vi "Device_Calibration.vi"(10 "PEU":refnum<class "PEU.lvclass">, 11 "E5071C":refnum<class "E5071C.lvclass">) -> ()   [LabVIEW 2020]
uses:
  Driver/E5071C/E5071C/E5071C.lvclass
  Driver/PEU/PEU/PEU.lvclass
panel:
  in  "TP1 - TP4":bool
  out ":SENS":i32
  in  "TP1 - TP3":bool
  in  "Next Button":bool
  in  "设置":bool
  in  "扫描点数":dbl=1001.0 caption="扫描点数\nSweep Points" min=2.0 max=1601.0 format="%#_6f"
  in  "中频带宽":dbl=70.0 caption="中频带宽\nIFBW" min=0.01 max=700.0 format="%#_6f kHz"
  in  "终止频率":dbl=20.0 caption="终止频率\nStop Frequency" min=0.0003 max=20.0 format="%#_6f GHz"
  in  "开始频率":dbl=300.0 caption="开始频率\nStart Frequency" min=300.0 max=20000000.0 format="%#_6f kHz"
  # "E5071C设置/校准"
  # "校准"
  # "参数设置"
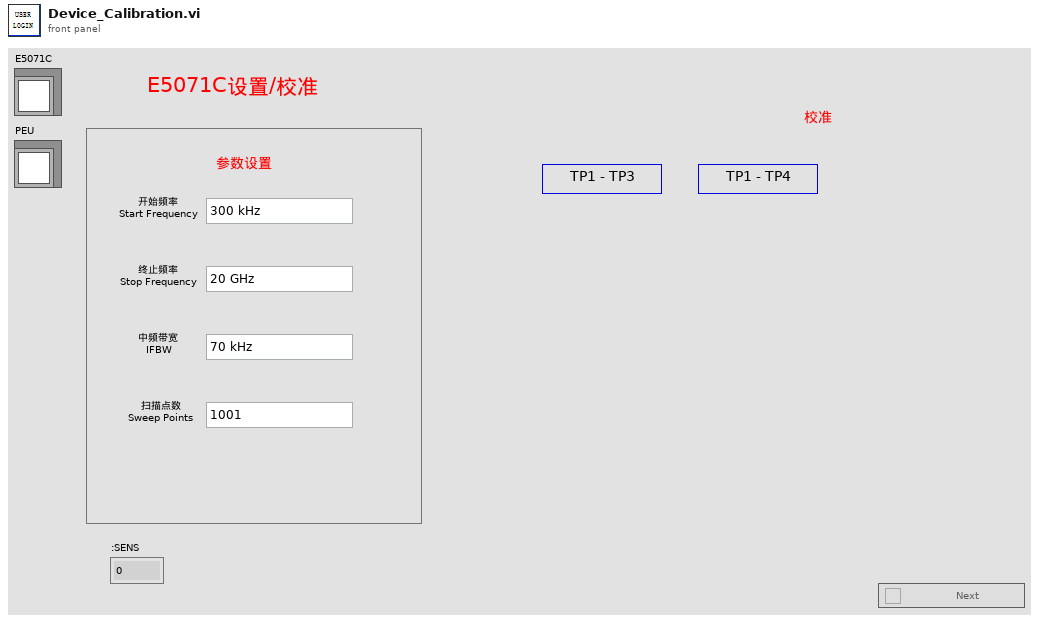
[diagram p1: front panel]
types:
  T1 = enum8{"Enabled", "Disabled", "Disabled and Grayed Out"}
  T2 = cluster{"E5071C":refnum<class "E5071C.lvclass">, "TP":string, "TPs":string[], "PEU":refnum<class "PEU.lvclass">}
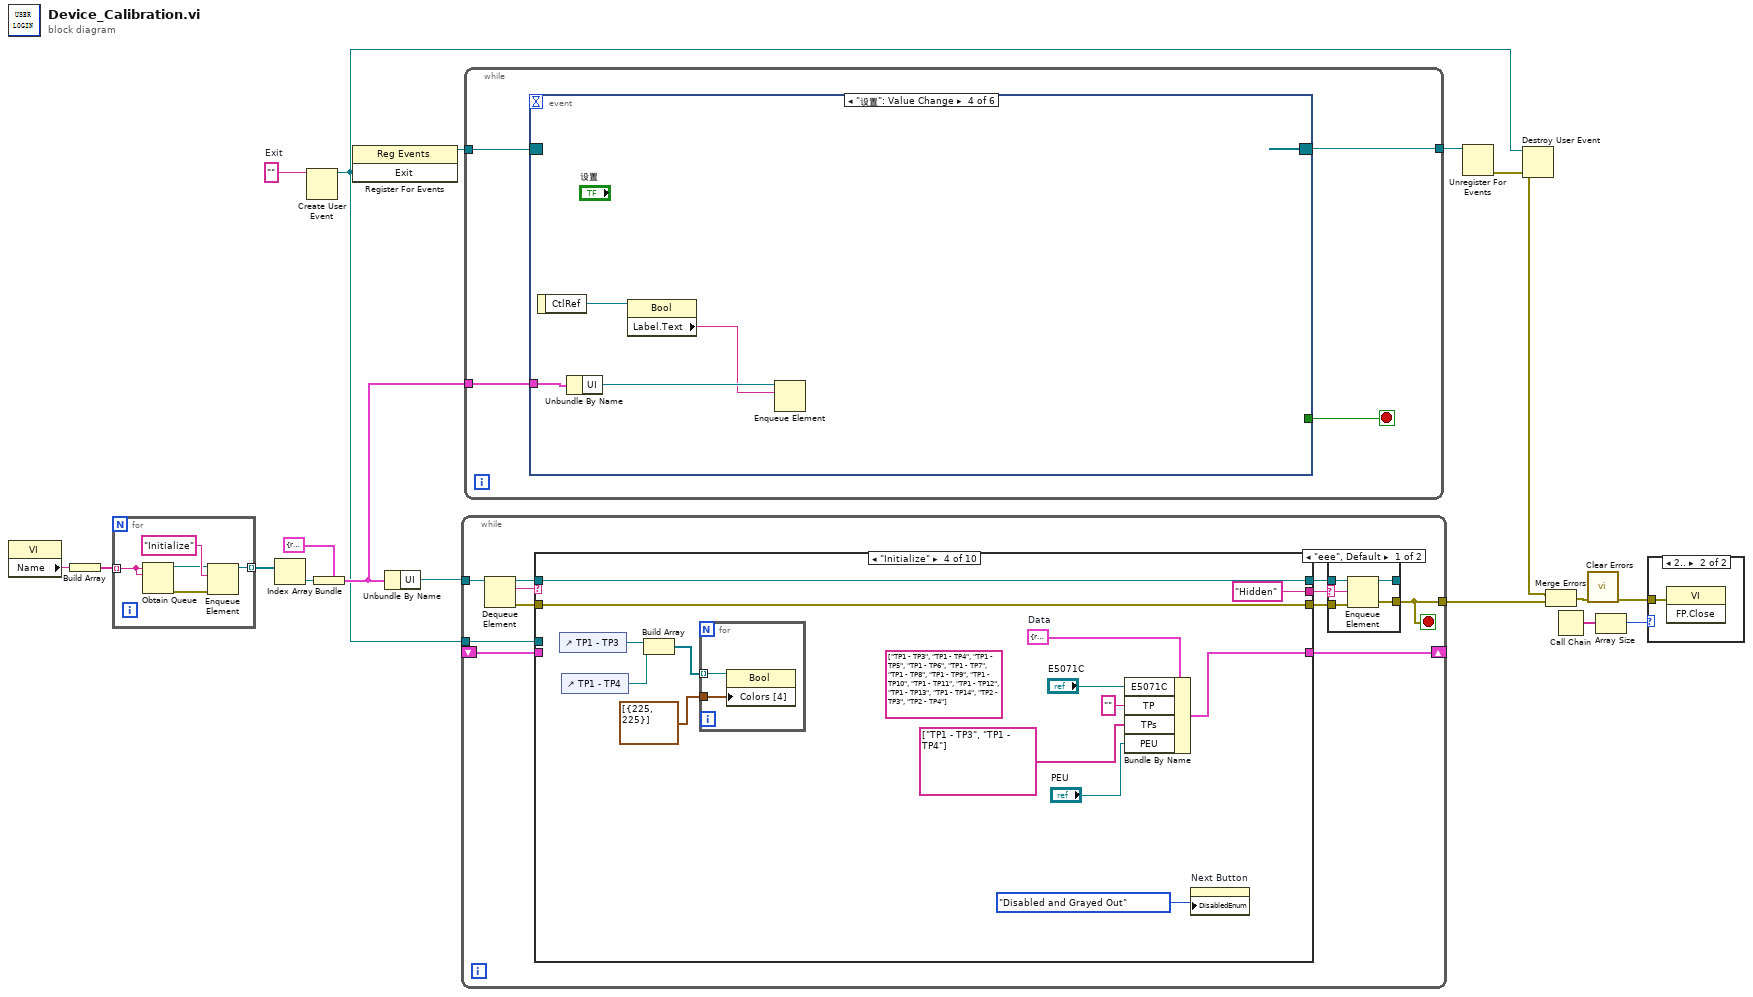
[diagram p0: block diagram]
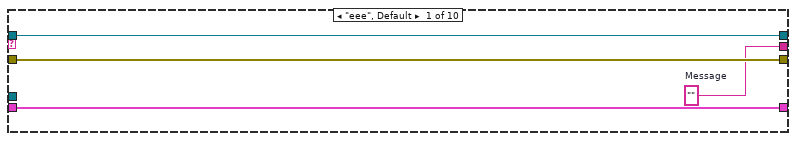
[diagram p4: hidden frame]
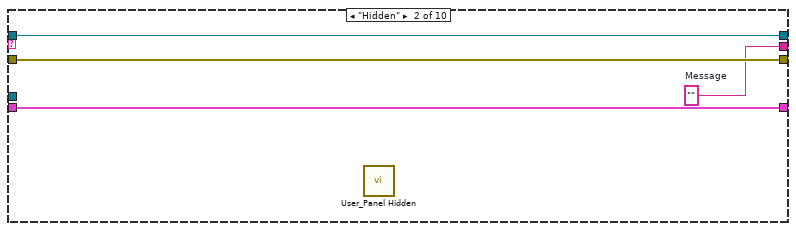
[diagram p5: hidden frame]
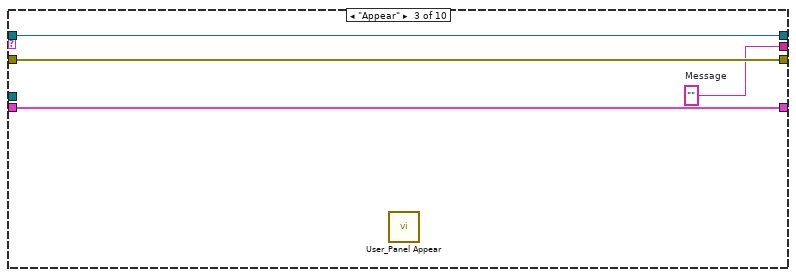
[diagram p6: hidden frame]
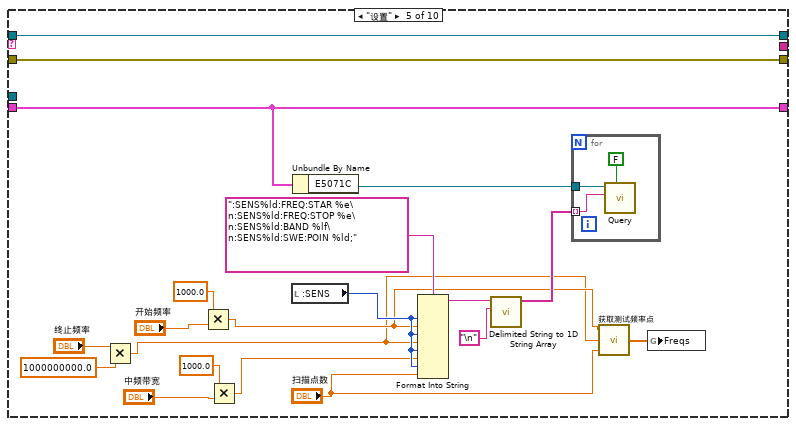
[diagram p7: hidden frame]
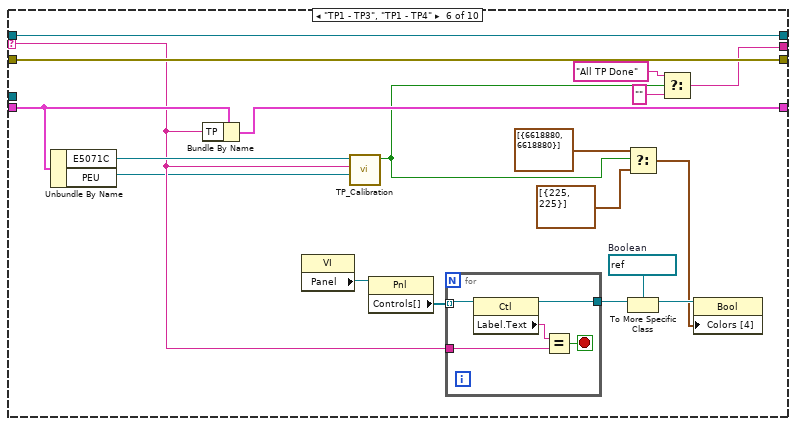
[diagram p8: hidden frame]
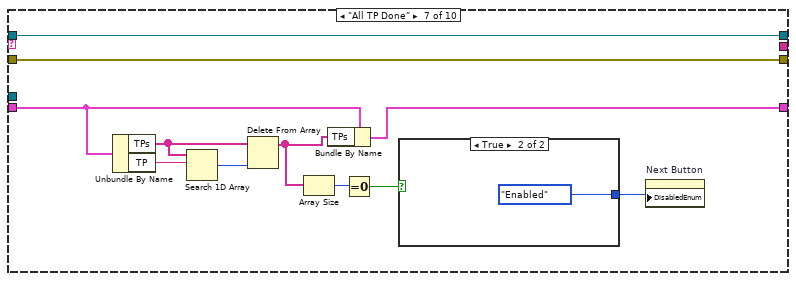
[diagram p9: hidden frame]
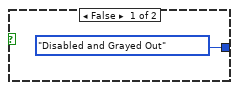
[diagram p10: hidden frame]
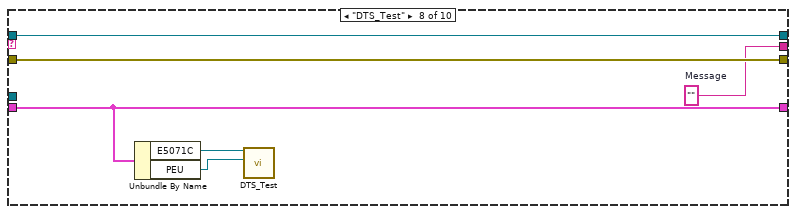
[diagram p11: hidden frame]
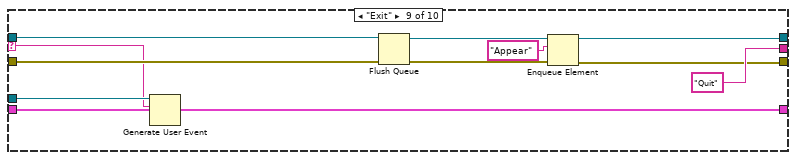
[diagram p12: hidden frame]
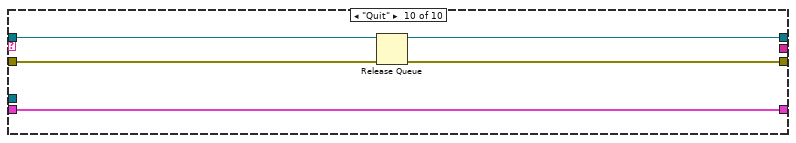
[diagram p13: hidden frame]
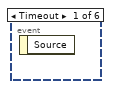
[diagram p14: hidden frame]
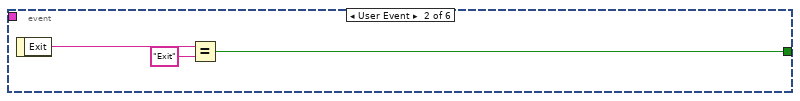
[diagram p15: hidden frame]
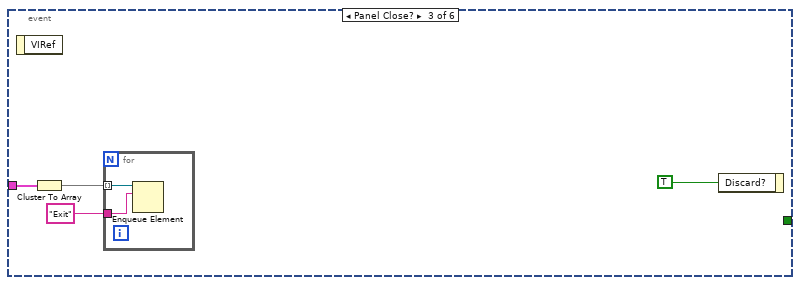
[diagram p16: hidden frame]
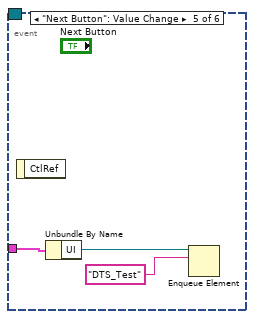
[diagram p17: hidden frame]
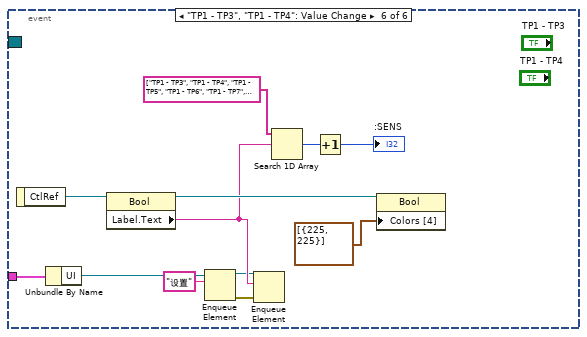
[diagram p18: hidden frame]
diagram:
  w7 = ""  # Exit
  n1 = property class="VI"() -> ("Name"=w17:string)  [unwired: 2 in, 2 out]
  n2 = Build Array(w17) -> (w18:string[])
  n3 = for {
    tunnel: w18 -> [w19] mode=indexing
    tunnel: [w20] -> w12 mode=indexing
    n4 = Obtain Queue(name (unnamed)=w19, element data type=w19) -> (queue out=w22:refnum<queue>, error out=w21:errorcluster)  [unwired: 3 in, 1 out]
    n5 = Enqueue Element(queue=w22, element="Initialize" ("元素"), error in (no error)=w21) -> (queue out=w20:refnum<queue>)  [unwired: 1 in, 2 out]
  }
  n6 = Index Array(array=w12) -> (element=w15:refnum<queue>)  [unwired: 1 in]
  n7 = Create User Event(user event datatype=w7) -> (user event=w11:refnum<user-event>)  [unwired: 1 in, 1 out]
  n8 = Bundle(cluster=cluster{"UI":refnum<queue>} {"UI"=refnum}, "UI"=w15) -> (w16:cluster{"UI":refnum<queue>})
  n9 = register-events(w11) -> (reference out=w8:refnum<event-registration>)  [unwired: 2 in, 1 out]
  n10 = Unbundle By Name(w16) -> ("UI"=w13:refnum<queue>)
  n11 = while {
    tunnel: w13 -> [w34]
    tunnel: [w24] -> w1
    shift-right: [w28] -> _
    shift-left: _ -> [w27]
    tunnel: w11 -> [w26]
    stop <- w24 stop-if-true
    n12 = Dequeue Element(queue=w34) -> (queue out=w33:refnum<queue>, element=w25:string, error out=w30:errorcluster)  [unwired: 2 in, 1 out]
    n13 = case shown="\"Initialize\"" w25 {
      selector: w25 -> [_ _ _ _ _ w99 _ _ w141 _]
      tunnel: w33 -> [w45 w49 w53 w67 w89 w111 w127 w135 w144 w150]
      tunnel: [w45 w49 w53 w67 w89 w111 w127 w135 w136 w150] -> w32
      tunnel: [w44 w48 w52 w66 w88 w110 w126 w134 w137 w147] -> w31
      tunnel: w30 -> [w44 w48 w52 w66 w88 w110 w126 w134 w143 w149]
      tunnel: [w43 w47 w51 "Hidden" ("Message") _ w95 _ w133 "Quit" ("Message") _] -> w29
      tunnel: [w42 w46 w50 w63 w87 w98 w119 w132 w146 w148] -> w28
      tunnel: w27 -> [w42 w46 w50 _ w87 w100 w121 w132 w146 w148]
      tunnel: w26 -> [_ _ _ _ _ _ _ _ w142 _]
      frame "eee", Default {
        w43 = ""  # Message
      }
      frame "Hidden" {
        w47 = ""  # Message
        n14 = call "User_Panel Hidden.vi"() -> ()  [unwired: 11 in, 1 out]
      }
      frame "Appear" {
        w51 = ""  # Message
        n15 = call "User_Panel Appear.vi"() -> ()  [unwired: 11 in, 1 out]
      }
      frame "Initialize" {
        (unwired) string[] ["TP1 - TP3", "TP1 - TP4", "TP1 - TP5", "TP1 - TP6", "TP1 - TP7", "TP1 - TP8", "TP1 - TP9", "TP1 - TP10", "TP1 - TP11", "TP1 - TP12", "TP1 - TP13", "TP1 - TP14", "TP2 - TP3", "TP2 - TP4"]
        w65 = T2 {"E5071C"=refnum, "TP"="", "TPs"=["TP1 - TP3", "TP1 - TP4", "TP1 - TP5", "TP1 - TP6", "TP1 - TP7", "TP1 - TP8", "TP1 - TP9", "TP1 - TP10", "TP1 - TP11", "TP1 - TP12", "TP1 - TP13", "TP1 - TP14", "TP2 - TP3", "TP2 - TP4"], "PEU"=refnum}  # Data
        n16 = control-ref of="TP1 - TP3"() -> (w55:refnum<vi>)
        n17 = control-ref of="TP1 - TP4"() -> (w56:refnum<vi>)
        n18 = Build Array(w55, w56) -> (w58:refnum<vi>[])
        n19 = for {
          tunnel: w58 -> [w69] mode=indexing
          tunnel: cluster{u32, u32}[] [{225, 225}] ("Colors [4]") -> [w68]
          n20 = property class="Bool"(reference=w69, "Colors [4]"=w68) -> ()  [unwired: 1 in, 2 out]
        }
        n21 = Bundle By Name(cluster=w65, "E5071C"="E5071C", "TP"="", "TPs"=string[] ["TP1 - TP3", "TP1 - TP4"], "PEU"="PEU") -> (w63:T2)
        n22 = property on="Next Button" class="Bool"("DisabledEnum"=T1."Disabled and Grayed Out" ("Disabled")) -> ()  [unwired: 2 in, 2 out]
      }
      frame "设置" {
        n23 = Multiply(x="终止频率", y=1000000000.0) -> (x*y=w72:dbl)
        n24 = Multiply(x=1000.0, y="开始频率") -> (x*y=w73:dbl)
        n25 = Multiply(x=1000.0, y="中频带宽") -> (x*y=w74:dbl)
        n26 = local read ":SENS"() -> (w81:i32)
        n27 = Unbundle By Name(w87) -> ("E5071C"=w86:refnum<class "E5071C.lvclass">)
        n28 = Format Into String(format string=":SENS%ld:FREQ:STAR %e\n:SENS%ld:FREQ:STOP %e\n:SENS%ld:BAND %lf\n:SENS%ld:SWE:POIN %ld;", w81, w73, w81, w72, w81, w74, w81, "扫描点数") -> (resulting string=w84:string)  [unwired: 2 in, 1 out]
        n29 = call <vilib>:"Delimited String to 1D String Array.vi"("delimiter"="\n", "delimited string"=w84) -> ("string array"=w82:string[])  [unwired: 9 in]
        n30 = for {
          tunnel: w86 -> [w92]
          tunnel: w82 -> [w90] mode=indexing
          n31 = call "Query.vi"("Return"=FALSE, "Command"=w90, "E5071C in"=w92) -> ()  [unwired: 6 in, 3 out]
        }
        n32 = call "获取测试频率点.vi"("测量点数"="扫描点数", "终止频率"=w72, "起始频率"=w73) -> ("Freq"=w70:dbl[])
        n33 = global write "Global.vi" "Freqs"(w70) -> ()
      }
      frame "TP1 - TP3", "TP1 - TP4" {
        w106 = refnum<vi> refnum  # Boolean
        n34 = Unbundle By Name(w100) -> ("E5071C"=w109:refnum<class "E5071C.lvclass">, "PEU"=w93:refnum<class "PEU.lvclass">)
        n35 = Bundle By Name(cluster=w100, "TP"=w99) -> (w98:T2)
        n36 = property class="VI"() -> ("Panel"=w108:refnum<vi>)  [unwired: 2 in, 2 out]
        n37 = call "TP_Calibration.vi"("PEU"=w93, "TP"=w99, "E5071C"=w109) -> ("Calibration Done"=w97:bool)  [unwired: 8 in]
        n38 = property class="Pnl"(reference=w108) -> ("Controls[]"=w107:refnum<vi>[])  [unwired: 1 in, 2 out]
        n39 = for {
          tunnel: w107 -> [w116] mode=indexing
          tunnel: w99 -> [w114]
          tunnel: [w112] -> w105
          stop <- w113 stop-if-true
          n40 = property class="Ctl"(reference=w116) -> (reference out=w112:refnum<vi>, "Label.Text"=w115:string)  [unwired: 1 in, 1 out]
          n41 = Equal?(x=w115, y=w114) -> (x = y?=w113:bool)
        }
        n42 = Select(t=cluster{u32, u32}[] [{6618880, 6618880}] ("Colors [4]"), s=w97, f=cluster{u32, u32}[] [{225, 225}] ("Colors [4]")) -> (s? t:f=w101:cluster{u32, u32}[])
        n43 = To More Specific Class(target class=w106, reference=w105) -> (specific class reference=w104:refnum<vi>)  [unwired: 1 in, 1 out]
        n44 = Select(t="All TP Done" ("Message"), s=w97, f="") -> (s? t:f=w95:string)
        n45 = property class="Bool"(reference=w104, "Colors [4]"=w101) -> ()  [unwired: 1 in, 2 out]
      }
      frame "All TP Done" {
        n46 = Unbundle By Name(w121) -> ("TPs"=w124:string[], "TP"=w125:string)
        n47 = Search 1D Array(1D array=w124, element=w125) -> (index of element=w123:i32)  [unwired: 1 in]
        n48 = Delete From Array(array=w124, index=w123) -> (array with subset deleted=w120:string[])  [unwired: 1 in, 1 out]
        n49 = Array Size(array=w120) -> (size(s)=w122:i32)
        n50 = Bundle By Name(cluster=w121, "TPs"=w120) -> (w119:T2)
        n51 = Equal To 0?(x=w122) -> (x = 0?=w118:bool)
        n52 = case shown="True" w118 {
          tunnel: [T1."Disabled and Grayed Out" ("Disabled") T1."Enabled" ("Disabled")] -> w117
          frame False {
          }
          frame True {
          }
        }
        n53 = property on="Next Button" class="Bool"("DisabledEnum"=w117) -> ()  [unwired: 2 in, 2 out]
      }
      frame "DTS_Test" {
        w133 = ""  # Message
        n54 = Unbundle By Name(w132) -> ("E5071C"=w131:refnum<class "E5071C.lvclass">, "PEU"=w130:refnum<class "PEU.lvclass">)
        n55 = call "DTS_Test.vi"("PEU"=w130, "E5071C"=w131) -> ()  [unwired: 10 in]
      }
      frame "Exit" {
        n56 = Generate User Event(user event=w142, event data cluster=w141) -> ()  [unwired: 2 in, 2 out]
        n57 = Flush Queue(queue=w144, error in (no error)=w143) -> (queue out=w139:refnum<queue>, error out=w138:errorcluster)  [unwired: 1 out]
        n58 = Enqueue Element(queue=w139, element="Appear" ("元素"), error in (no error)=w138) -> (queue out=w136:refnum<queue>, error out=w137:errorcluster)  [unwired: 1 in, 1 out]
      }
      frame "Quit" {
        n59 = Release Queue(queue=w150, error in (no error)=w149) -> (error out=w147:errorcluster)  [unwired: 1 in, 2 out]
      }
    }
    n60 = case shown="\"eee\", Default" w29 {
      selector: w29 -> [w35 _]
      tunnel: w32 -> [w39 w41]
      tunnel: w31 -> [w38 w40]
      tunnel: [w37 w40] -> w24
      tunnel: [w36 w41] -> _
      frame "eee", Default {
        n61 = Enqueue Element(queue=w39, element=w35, error in (no error)=w38) -> (queue out=w36:refnum<queue>, error out=w37:errorcluster)  [unwired: 1 in, 1 out]
      }
      frame "" {
      }
    }
  }
  n62 = while {
    tunnel: w8 -> [w153]
    tunnel: [w152] -> w10
    tunnel: w16 -> [w151]
    stop <- w154 stop-if-true
    n63 = event shown="[3] \"设置\": Value Change" {
      selector: w153 -> [_ _ _ _ _ _]
      dyn-events: [_ _ _ _ _ _] -> w152
      timeout: _ -> [_ _ _ _ _ _]
      tunnel: [_ w156 _ _ _ _] -> w154
      tunnel: w151 -> [_ _ w160 w165 w169 w182]
      event Timeout {
        n64 = event-data() -> ()  [unwired: 1 in, 1 out]
      }
      event User Event {
        n65 = event-data() -> ("Exit"=w157:string)  [unwired: 1 in]
        n66 = Equal?(x=w157, y="Exit") -> (x = y?=w156:bool)
      }
      event Panel Close? {
        n67 = event-data() -> ()  [unwired: 1 in, 1 out]
        n68 = Cluster To Array(cluster=w160) -> (array=w159:refnum<queue>[])
        n69 = for {
          tunnel: w159 -> [w163] mode=indexing
          tunnel: "Exit" ("元素") -> [w162]
          n70 = Enqueue Element(queue=w163, element=w162) -> ()  [unwired: 2 in, 3 out]
        }
        n71 = event-data("Discard?"=TRUE ("放弃？")) -> ()  [unwired: 1 in, 1 out]
      }
      event "设置": Value Change {
        n72 = event-data() -> ("CtlRef"=w164:refnum<vi>)  [unwired: 1 in]
        n73 = Unbundle By Name(w165) -> ("UI"=w167:refnum<queue>)
        n74 = property class="Bool"(reference=w164) -> ("Label.Text"=w166:string)  [unwired: 1 in, 2 out]
        n75 = Enqueue Element(queue=w167, element=w166) -> ()  [unwired: 2 in, 3 out]
      }
      event "Next Button": Value Change {
        n76 = event-data() -> ()  [unwired: 1 in, 1 out]
        n77 = Unbundle By Name(w169) -> ("UI"=w170:refnum<queue>)
        n78 = Enqueue Element(queue=w170, element="DTS_Test") -> ()  [unwired: 2 in, 3 out]
      }
      event "TP1 - TP3", "TP1 - TP4": Value Change {
        n79 = event-data() -> ("CtlRef"=w181:refnum<vi>)  [unwired: 1 in]
        n80 = Unbundle By Name(w182) -> ("UI"=w175:refnum<queue>)
        n81 = property class="Bool"(reference=w181) -> (reference out=w180:refnum<vi>, "Label.Text"=w177:string)  [unwired: 1 in, 1 out]
        n82 = Enqueue Element(queue=w175, element="设置") -> (queue out=w174:refnum<queue>, error out=w173:errorcluster)  [unwired: 2 in, 1 out]
        n83 = Enqueue Element(queue=w174, element=w177, error in (no error)=w173) -> ()  [unwired: 1 in, 3 out]
        n84 = Search 1D Array(1D array=string[] ["TP1 - TP3", "TP1 - TP4", "TP1 - TP5", "TP1 - TP6", "TP1 - TP7", "TP1 - TP8", "TP1 - TP9", "TP1 - TP10", "TP1 - TP11", "TP1 - TP12", "TP1 - TP13", "TP1 - TP14", "TP2 - TP3", "TP2 - TP4"], element=w177) -> (index of element=w176:i32)  [unwired: 1 in]
        n85 = Increment(x=w176) -> (x+1=→":SENS":i32)
        n86 = property class="Bool"(reference=w180, "Colors [4]"=cluster{u32, u32}[] [{225, 225}]) -> ()  [unwired: 1 in, 2 out]
      }
    }
  }
  n87 = Unregister For Events(event registration refnum=w10) -> (error out=w9:errorcluster)  [unwired: 1 in]
  n88 = Destroy User Event(user event=w11, error in=w9) -> (error out=w2:errorcluster)
  n89 = Merge Errors(w2, w1) -> (w6:errorcluster)
  n90 = Call Chain() -> (call chain=w4:string[])
  n91 = call <vilib>:"Clear Errors.vi"("error in (no error)"=w6) -> ("error out"=w5:errorcluster)  [unwired: 5 in, 1 out]
  n92 = Array Size(array=w4) -> (size(s)=w3:i32)
  n93 = case shown="2.." w3 {
    tunnel: w5 -> [_ w183]
    frame 0, Default {
    }
    frame 2.. {
      n94 = invoke class="VI" method="FP.Close"(error in=w183) -> ()  [unwired: 2 in, 3 out]
    }
  }
